vi "Set Data.vi"(8 "error in (no error)":errorcluster, 10 "Data":cluster{"Error":sgl, "# of Obs":u16}, 11 "Stability Data in":refnum<class "Stability Data.lvclass">) -> (0 "error out":errorcluster, 3 "Stability Data out":refnum<class "Stability Data.lvclass">)   [LabVIEW 2015, in "Stability Data.lvclass"]
uses:
  Stability Data.lvclass
  Stability Data.lvclass/Stability Data.ctl
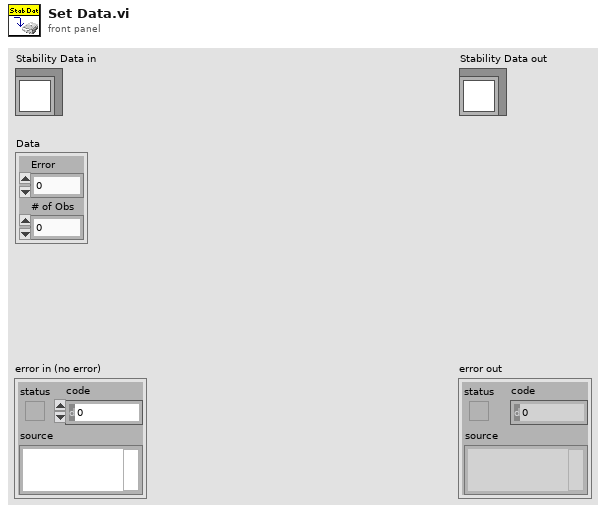
[diagram p1: front panel]
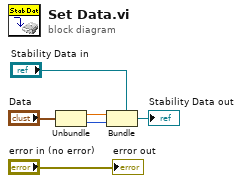
[diagram p0: block diagram]
diagram:
  n1 = Unbundle("Data") -> ("Error"=w2:sgl, "# of Obs"=w1:u16)
  n2 = Bundle(cluster="Stability Data in", w2, w1) -> (→"Stability Data out":refnum<class "Stability Data.lvclass">)
  "error out" <- "error in (no error)"
